vi "TestExec.Run Executable and Parse Results V1.vi"(4 "SuppressActionReport":bool, 6 "Reset":bool, 7 "Vars":variant, 8 "error in":errorcluster, 9 "Timeout(s)":dbl=500.0 caption="Time Out(s)" format="%.2f", 10 "Output Folder":path, 11 "Utility Config File":path) -> (0 "Error":errorcluster, 3 "RTN Data":T1 {"MeasData"."Status" items=["LOG", "PASS", "FAIL", "ERROR"]; "Attr"."Status" items=["LOG", "PASS", "FAIL", "ERROR"]; "Num"."Status" items=["LOG", "PASS", "FAIL", "ERROR"]})   [LabVIEW 2018]
uses:
  Cmd Exe/CmdExe.Output Error Check Setup.ctl
  Cmd Exe/CmdExe.Setup Params.ctl
  Results/Result.Measurement and Attribute Item Status.ctl
  Results/Result.Attribute.ctl
  Results/Result.Limit Type.ctl
  Results/Result.Numeric.ctl
  Results/Result XML/TestResult.SW Item.ctl
  Reports/Report.Result FileDataObject.ctl
  TestExec.Local Result Data.ctl
  <vilib>/KATE/Time/Time Utils.lvlib
  Results/Result.Measurement Item.ctl
panel:
  in  "Tab Control":enum32{"Execute", "Results"}(tab)
  out "Active":bool
  out "Sys Exec Commands":string
  out "Sys Exec STDOut":string
  out "Dur(s)":dbl caption="Duration(s)" format="%.3f"
  out "Rslt":u32(colorbox)=13816530 caption="Exe"
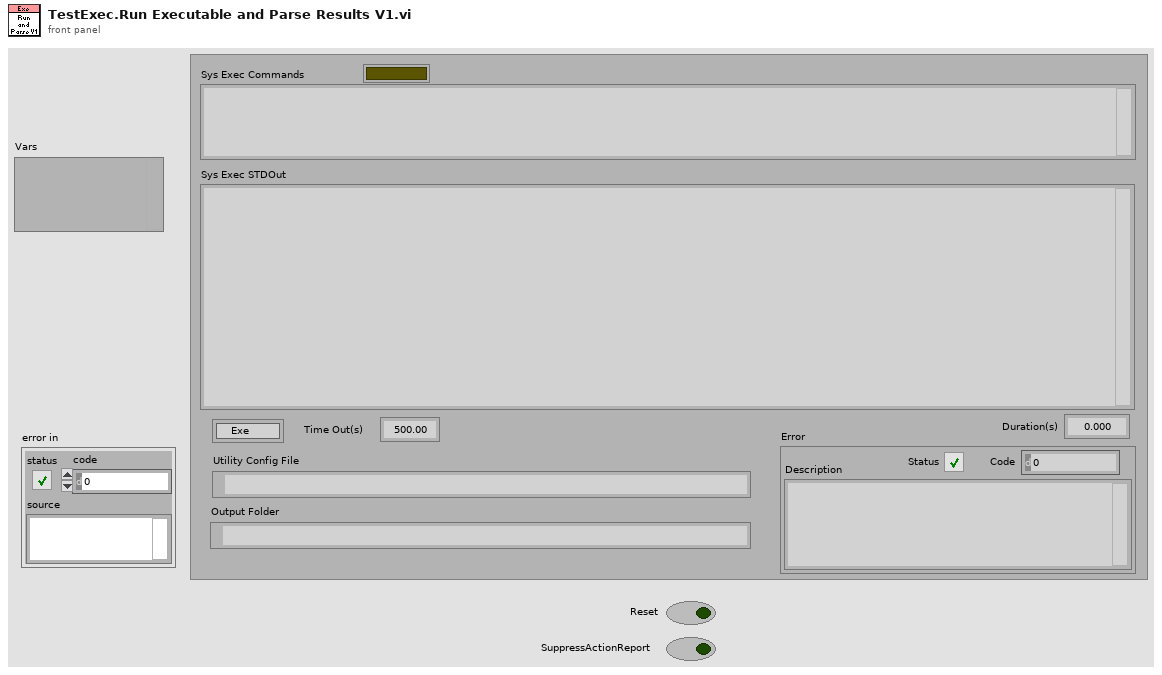
[diagram p1: front panel]
types:
  T1 = typedef "TestExec.Local Result Data.ctl" = cluster{"Attr":T2[], "Num":T4[], "UUT Props":string[][], "Vars":string[][], "SW Items":T6[], "Error":errorcluster, "Step":i32, "FileObjs":T7[], "MeasData":T8[]}
  T2 = typedef "Result.Attribute.ctl" = cluster{"Cnt":i32, "Step":string, "Category":string, "Name":string, "Value":string, "Status":T3, "Code":i32, "Desc":string, "Time":timestamp}
  T3 = typedef "Result.Measurement and Attribute Item Status.ctl" = i32
  T4 = typedef "Result.Numeric.ctl" = cluster{"Cnt":i32, "Step":string, "Category":string, "Name":string, "Value":dbl, "Units":string, "LimType":T5, "LL":dbl, "UL":dbl, "Status":T3, "Code":i32, "Desc":string, "Time":timestamp}
  T5 = typedef "Result.Limit Type.ctl" = enum16{"None", "EQ", "NE", "GT", "LT", "GE", "LE", "GTLT", "GELE", "GELT", "GTLE", "LTGT", "LEGE", "LEGT", "LTGE", "Contains", "NotContains"}
  T6 = typedef "TestResult.SW Item.ctl" = cluster{"Name":string, "PN":string, "Version":string, "Note":string}
  T7 = typedef "Report.Result FileDataObject.ctl" = cluster{"Cnt":i32, "Step":string, "Category":string, "Name":string, "Type":string, "File Name":string, "Time":string, "Path":path}
  T8 = typedef "Result.Measurement Item.ctl" = cluster{"Cnt":i32, "Step":string, "Category":string, "Name":string, "Value":string, "Units":string, "LimType":string, "LL":string, "UL":string, "Status":T3, "Code":i32, "Desc":string, "Time":timestamp}
  T9 = typedef "CmdExe.Setup Params.ctl" = cluster{"Timeout (s)":dbl, "Show Cmd Win":bool, "Error Check":T10, "Log_En":bool, "LogFileName":string, "LogDir":path}
  T10 = typedef "CmdExe.Output Error Check Setup.ctl" = cluster{"StdOut_Ck":bool, "StdOutErrMsgs":string[], "StdErr_Ck":bool, "RtnCode_Ck":bool, "RtnCodePASS":i32}
  T11 = cluster{"Args":string, "Setup":T9, "StdOut":string, "ActionName":string, "Exe":path, "RTN Data":T1, "Prefix":string, "Code":i32}
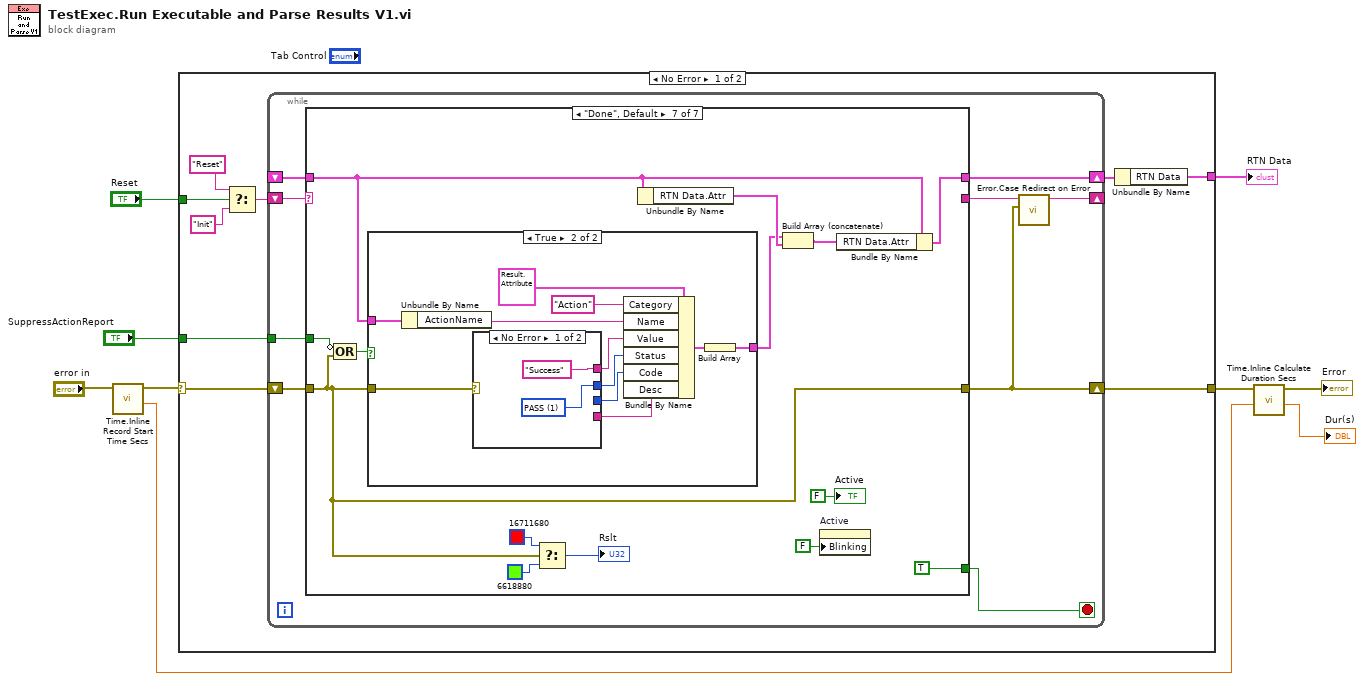
[diagram p0: block diagram]
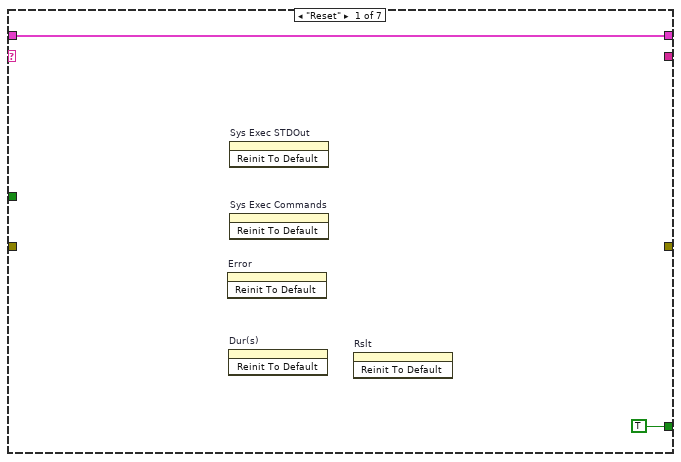
[diagram p2: hidden frame]
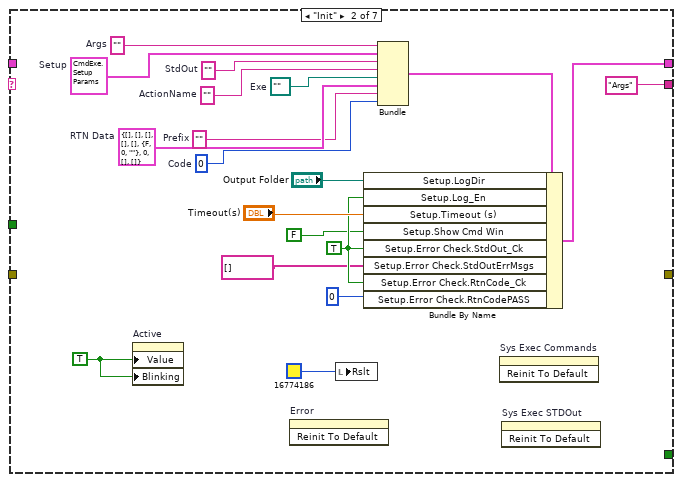
[diagram p3: hidden frame]
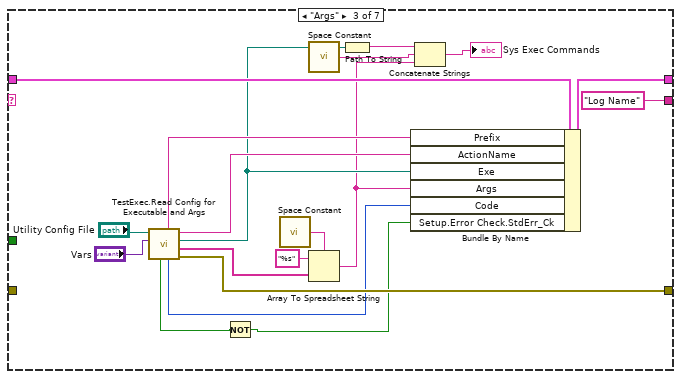
[diagram p4: hidden frame]
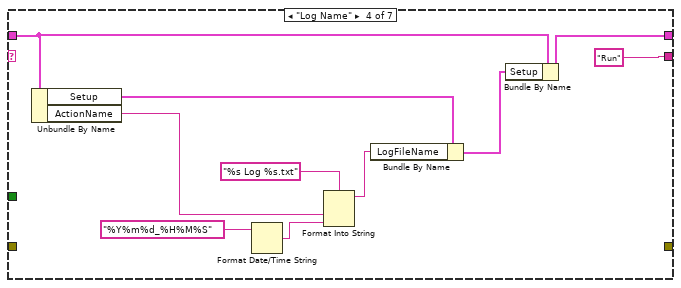
[diagram p5: hidden frame]
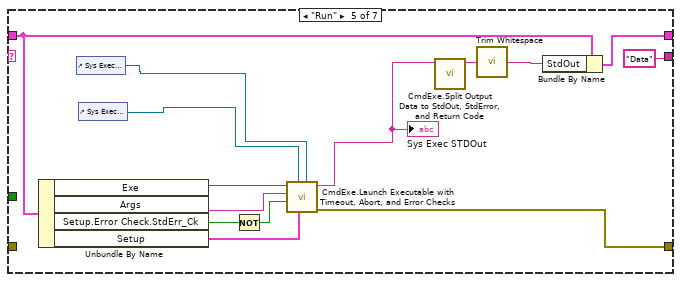
[diagram p6: hidden frame]
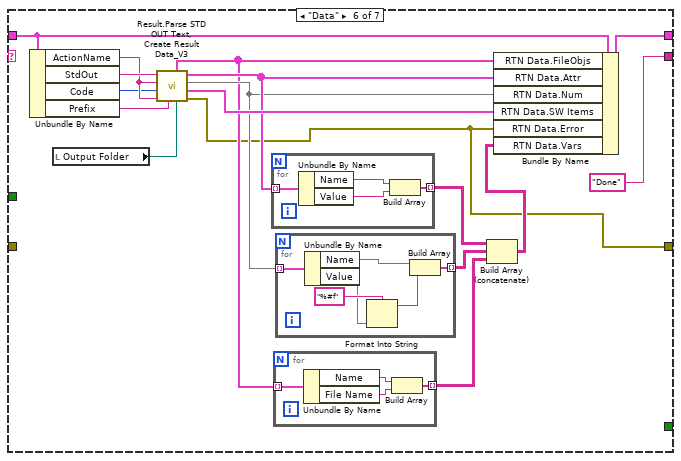
[diagram p7: hidden frame]
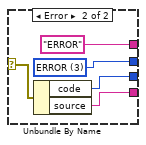
[diagram p9: hidden frame]
diagram:
  n1 = call <vilib>:"Time.Inline Record Start Time Secs.vi"("Error In Upper"="error in") -> ("Start(s)"=w3:dbl, "Error Out Upper"=w7:errorcluster)  [unwired: 8 in, 1 out]
  n2 = case shown="No Error" w7 {
    selector: w7 -> [w18 w155]
    tunnel: [w17 w155] -> w5
    tunnel: [w15 _] -> w9
    tunnel: "Reset" -> [w11 _]
    tunnel: "SuppressActionReport" -> [w10 _]
    frame No Error {
      n3 = Select(t="Reset", s=w11, f="Init") -> (s? t:f=w13:string)
      n4 = while {
        shift-right: [w21] -> _
        shift-left: w13 -> [w27]
        shift-right: [w26] -> w16
        shift-left: _ -> [w25]
        shift-right: [w20] -> w17
        shift-left: w18 -> [w23]
        tunnel: w10 -> [w19]
        stop <- w24 stop-if-true
        n5 = case shown="\"Done\", Default" w27 {
          tunnel: [_ "Args" "Log Name" "Run" "Data" "Done" _] -> w22
          tunnel: [w29 w40 w67 w76 w81 w105 w127] -> w26
          tunnel: w25 -> [w29 _ w66 w75 w83 w104 w126]
          tunnel: [TRUE _ _ _ _ _ TRUE] -> w24
          tunnel: w23 -> [_ _ _ _ _ _ w125]
          tunnel: [_ _ w59 _ w80 w94 w125] -> w20
          tunnel: w19 -> [_ _ _ _ _ _ w124]
          frame "Reset" {
            n6 = invoke on="Error" class="Clust (strict)" method="Reinit To Default"() -> ()  [unwired: 3 in, 3 out]
            n7 = invoke on="Dur(s)" class="DigNum (strict)" method="Reinit To Default"() -> ()  [unwired: 3 in, 3 out]
            n8 = invoke on="Sys Exec STDOut" class="Str" method="Reinit To Default"() -> ()  [unwired: 3 in, 3 out]
            n9 = invoke on="Sys Exec Commands" class="Str" method="Reinit To Default"() -> ()  [unwired: 3 in, 3 out]
            n10 = invoke on="Rslt" class="ColBox" method="Reinit To Default"() -> ()  [unwired: 3 in, 3 out]
          }
          frame "Init" {
            w30 = 0  # Code
            w31 = ""  # Prefix
            w32 = T1 {"Attr"=[], "Num"=[], "UUT Props"=[], "Vars"=[], "SW Items"=[], "Error"={"status"=FALSE, "code"=0, "source"=""}, "Step"=0, "FileObjs"=[], "MeasData"=[]}  # RTN Data
            w33 = path ""  # Exe
            w34 = ""  # ActionName
            w37 = ""  # StdOut
            w41 = TRUE
            w46 = TRUE ("Value")
            w45 = T9 {"Timeout (s)"=60.0, "Show Cmd Win"=FALSE, "Error Check"={"StdOut_Ck"=FALSE, "StdOutErrMsgs"=["Error", "Unable to find device "], "StdErr_Ck"=FALSE, "RtnCode_Ck"=FALSE, "RtnCodePASS"=0}, "Log_En"=FALSE, "LogFileName"="", "LogDir"=path ""}  # Setup
            w48 = ""  # Args
            n11 = property on="Active" class="Bool (strict)"("Value"=w46, "Blinking"=w46) -> ()  [unwired: 2 in, 2 out]
            n12 = invoke on="Error" class="Clust (strict)" method="Reinit To Default"() -> ()  [unwired: 3 in, 3 out]
            n13 = local write "Rslt"(u32 16774186) -> ()
            n14 = Bundle("Args"=w48, "Setup"=w45, "StdOut"=w37, "ActionName"=w34, "Exe"=w33, "RTN Data"=w32, "Prefix"=w31, "Code"=w30) -> (w42:T11)  [unwired: 1 in]
            n15 = Bundle By Name(cluster=w42, "Setup.LogDir"="Output Folder", "Setup.Log_En"=w41, "Setup.Timeout (s)"="Timeout(s)", "Setup.Show Cmd Win"=FALSE, "Setup.Error Check.StdOut_Ck"=w41, "Setup.Error Check.StdOutErrMsgs"=string[] [], "Setup.Error Check.RtnCode_Ck"=w41, "Setup.Error Check.RtnCodePASS"=0 ("Error Check.RtnCodePASS")) -> (w40:T11)
            n16 = invoke on="Sys Exec Commands" class="Str" method="Reinit To Default"() -> ()  [unwired: 3 in, 3 out]
            n17 = invoke on="Sys Exec STDOut" class="Str" method="Reinit To Default"() -> ()  [unwired: 3 in, 3 out]
          }
          frame "Args" {
            n18 = call "TestExec.Read Config for Executable and Args.vi"("Vars"="Vars", "Config File"="Utility Config File") -> ("error out"=w59:errorcluster, "Args"=w61:string[], "Exe"=w53:path, "Action Name"=w58:string, "Error Code"=w57:i32, "Data Name Prefix"=w56:string, "IgnoreStdError"=w50:bool)  [unwired: 2 in, 1 out]
            n19 = Not(x=w50) -> (.not. x?=w49:bool)
            n20 = call <vilib>:"Space Constant.vi"() -> ("String"=w62:string)
            n21 = call <vilib>:"Space Constant.vi"() -> ("String"=w51:string)
            n22 = Array To Spreadsheet String(delimiter (Tab)=w62, array=w61, 3:"%s" ("format string")) -> (spreadsheet string=w52:string)
            n23 = Path To String(path=w53) -> (string=w54:string)
            n24 = Bundle By Name(cluster=w66, "Prefix"=w56, "ActionName"=w58, "Exe"=w53, "Args"=w52, "Code"=w57, "Setup.Error Check.StdErr_Ck"=w49) -> (w67:T11)
            n25 = Concatenate Strings(w54, w51, w52) -> (→"Sys Exec Commands":string)
          }
          frame "Log Name" {
            n26 = Unbundle By Name(w75) -> ("Setup"=w73:T9, "ActionName"=w68:string)
            n27 = Format Date/Time String(time format string (%c)="%Y%m%d_%H%M%S") -> (date/time string=w69:string)  [unwired: 2 in]
            n28 = Format Into String(format string="%s Log %s.txt", w68, w69) -> (resulting string=w70:string)  [unwired: 2 in, 1 out]
            n29 = Bundle By Name(cluster=w73, "LogFileName"=w70) -> (w74:T9)
            n30 = Bundle By Name(cluster=w75, "Setup"=w74) -> (w76:T11)
          }
          frame "Run" {
            n31 = Unbundle By Name(w83) -> ("Exe"=w82:path, "Args"=w91:string, "Setup.Error Check.StdErr_Ck"=w79:bool, "Setup"=w90:T9)
            n32 = control-ref of="Sys Exec Commands"() -> (w89:refnum<vi>)
            n33 = control-ref of="Sys Exec STDOut"() -> (w88:refnum<vi>)
            n34 = Not(x=w79) -> (.not. x?=w78:bool)
            n35 = call "CmdExe.Launch Executable with Timeout, Abort, and Error Checks.vi"("Cmd IN Ref"=w89, "Setup"=w90, "Output Ref"=w88, "Ignore StdErr"=w78, "Args"=w91, "Executable"=w82) -> ("error out"=w80:errorcluster, "Data Out"=w85:string)  [unwired: 2 in, 2 out]
            "Sys Exec STDOut" <- w85
            n36 = call "CmdExe.Split Output Data to StdOut, StdError, and Return Code.vi"("Output Data"=w85) -> ("StdOut"=w86:string)  [unwired: 7 in, 3 out]
            n37 = call <vilib>:"Trim Whitespace.vi"("string"=w86) -> ("trimmed string"=w84:string)  [unwired: 1 in]
            n38 = Bundle By Name(cluster=w83, "StdOut"=w84) -> (w81:T11)
          }
          frame "Data" {
            n39 = Unbundle By Name(w104) -> ("ActionName"=w100:string, "StdOut"=w108:string, "Code"=w93:i32, "Prefix"=w92:string)
            n40 = local read "Output Folder"() -> (w106:path)
            n41 = call "Result.Parse STD OUT Text, Create Result Data_V3.vi"("UUTDir"=w106, "Prefix"=w92, "Version Name"=w100, "Error Code"=w93, "Task Name"=w100, "StdOut"=w108) -> ("Error"=w94:errorcluster, "SW Ver"=w107:T6[], 2:w102, "Meas"=w103:T8[], "Data Files"=w101:T7[])  [unwired: 1 in]
            n42 = for {
              tunnel: w103 -> [w122] mode=indexing
              tunnel: [w119] -> w99 mode=indexing
              n43 = Unbundle By Name(w122) -> ("Name"=w121:string, "Value"=w120:string)
              n44 = Build Array(w121, w120) -> (w119:string[])
            }
            n45 = for {
              tunnel: w101 -> [w112] mode=indexing
              tunnel: [w110] -> w97 mode=indexing
              n46 = Unbundle By Name(w112) -> ("Name"=w111:string, "File Name"=w109:string)
              n47 = Build Array(w111, w109) -> (w110:string[])
            }
            n48 = for {
              tunnel: w102 -> [w118] mode=indexing
              tunnel: [w116] -> w98 mode=indexing
              n49 = Unbundle By Name(w118) -> ("Name"=w117, "Value"=w114)
              n50 = Format Into String(format string="%#f", w114) -> (resulting string=w113:string)  [unwired: 2 in, 1 out]
              n51 = Build Array(w117, w113) -> (w116:string[])
            }
            n52 = Build Array (concatenate)(w99, w98, w97) -> (w96:string[][])
            n53 = Bundle By Name(cluster=w104, "RTN Data.FileObjs"=w101, "RTN Data.Attr"=w103, "RTN Data.Num"=w102, "RTN Data.SW Items"=w107, "RTN Data.Error"=w94, "RTN Data.Vars"=w96) -> (w105:T11)
          }
          frame "Done", Default {
            n54 = Compound Arithmetic op=OR(invert w124, w125) -> (w123:bool)
            n55 = case shown="True" w123 {
              tunnel: [_ w140] -> w129
              tunnel: w126 -> [_ w139]
              tunnel: w125 -> [_ w137]
              frame False {
              }
              frame True {
                n56 = Unbundle By Name(w139) -> ("ActionName"=w138:string)
                n57 = case shown="No Error" w137 {
                  selector: w137 -> [_ w153]
                  tunnel: ["Success" "ERROR"] -> w145
                  tunnel: [w149 w150] -> w142
                  tunnel: [_ w152] -> w144
                  tunnel: [_ w151] -> w143
                  frame No Error {
                    w149 = T3 1 items=["LOG", "PASS", "FAIL", "ERROR"] ("Status")
                  }
                  frame Error {
                    w150 = T3 3 items=["LOG", "PASS", "FAIL", "ERROR"] ("Status")
                    n58 = Unbundle By Name(w153) -> ("code"=w152:i32, "source"=w151:string)
                  }
                }
                n59 = Bundle By Name(cluster=T2 {"Cnt"=0, "Step"="", "Category"="", "Name"="", "Value"="", "Status"=0, "Code"=0, "Desc"="", "Time"=timestamp(0 s since 1904-01-01)} ("Attribute"), "Category"="Action", "Name"=w138, "Value"=w145, "Status"=w142, "Code"=w144, "Desc"=w143) -> (w141:T2)
                n60 = Build Array(w141) -> (w140:T2[])
              }
            }
            n61 = Select(t=u32 16711680, s=w125, f=u32 6618880) -> (s? t:f=→"Rslt":u32)
            n62 = Unbundle By Name(w126) -> ("RTN Data.Attr"=w130:T2[])
            n63 = Build Array (concatenate)(w129, w130) -> (w131:T2[])
            n64 = property on="Active" class="Bool (strict)"("Blinking"=FALSE ("Value")) -> ()  [unwired: 2 in, 2 out]
            n65 = Bundle By Name(cluster=w126, "RTN Data.Attr"=w131) -> (w127:T11)
            "Active" <- FALSE ("Active")
          }
        }
        n66 = call "Error.Case Redirect on Error.vi"("error in"=w20, "Next Case"=w22) -> ("Next Case Out"=w21:string)  [unwired: 9 in]
      }
      n67 = Unbundle By Name(w16) -> ("RTN Data"=w15:T1)
    }
    frame Error {
    }
  }
  "RTN Data" <- w9
  n68 = call <vilib>:"Time.Inline Calculate Duration Secs.vi"("Start(Sec)"=w3, "Error In Top"=w5) -> ("Duration(s)"=→"Dur(s)":dbl, "Error Out Top"=→"Error":errorcluster)  [unwired: 7 in, 1 out]
